vi "CAN_Close.vi"(8 "error in (no error)":errorcluster caption="错误输入（无错误）", 11 "General_Input":T1) -> (0 "error out":errorcluster caption="错误输出", 3 "Closed":bool)   [LabVIEW 2012]
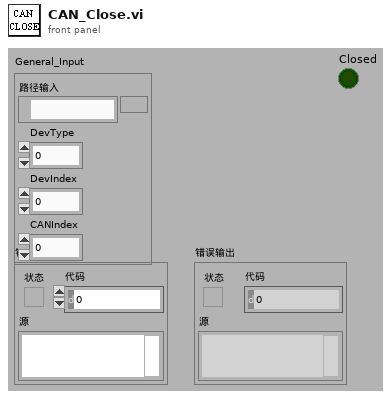
[diagram p1: front panel]
types:
  T1 = cluster{"路径输入":path, "DevType":u32, "DevIndex":u32, "CANIndex":u32}
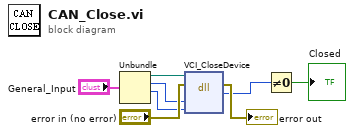
[diagram p0: block diagram]
diagram:
  n1 = Unbundle("General_Input") -> ("路径输入"=w5:path, "DevType"=w3:u32, "DevIndex"=w4:u32)  [unwired: 1 out]
  n2 = dll-call lib="?" fn="VCI_CloseDevice"(path in=w5, error in="error in (no error)", "DevType"=w3, "DevIndex"=w4) -> (error out=→"error out":errorcluster, "CloseOrNot"=w2:u32)  [unwired: 3 in, 1 out]
  n3 = Not Equal To 0?(x=w2) -> (x != 0?=→"Closed":bool)
